vi "Time Shift IG Array.vi"(1 "Time Since Last Shot":dbl=38319.99977827072 step=8.0 format="%<%H:%M:%S>t", 2 "IGvsTime Array":dbl[][](array[numeric])) -> (0 "IGvsTime TimeShifted":dbl[][](array[numeric]))   [LabVIEW 2016]
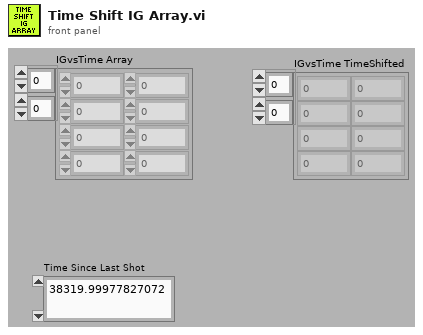
[diagram p1: front panel]
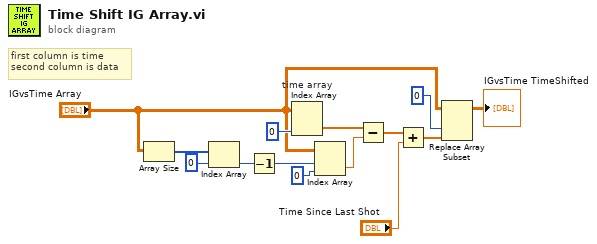
[diagram p0: block diagram]
diagram:
  # "first column is time\nsecond column is data"
  n1 = Array Size(array="IGvsTime Array") -> (size(s)=w14:i32[])
  n2 = Index Array(array=w14, index=0) -> (element=w11:i32)
  n3 = Decrement(x=w11) -> (x-1=w12:i32)
  n4 = Index Array "time array"(array="IGvsTime Array", index (col)=0 ("disabled index (col)")) -> (element=w2:dbl[])  [unwired: 1 in]
  n5 = Index Array(array="IGvsTime Array", index (row)=w12, index (col)=0 ("disabled index (col)")) -> (element=w1:dbl)
  n6 = Subtract(x=w2, y=w1) -> (x-y=w8:dbl[])
  n7 = Add(x=w8, y="Time Since Last Shot") -> (x+y=w5:dbl[])
  n8 = Replace Array Subset(array="IGvsTime Array", new element=w5, index (col)=0 ("disabled index (col)")) -> (→"IGvsTime TimeShifted":dbl[][])  [unwired: 1 in]
